vi "Read Com port Name.vi"(11 "Device in":refnum<class "PIC-Device.lvclass">) -> (2 "Com port Name":string, 3 "Device out":refnum<class "PIC-Device.lvclass">)   [LabVIEW 2020, in "PIC-Device.lvclass"]
uses:
  PIC-Device.lvclass
  PIC-Device.lvclass/PIC-Device.ctl
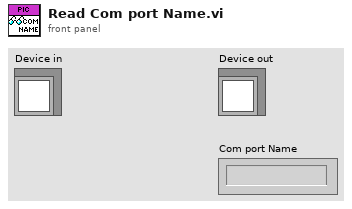
[diagram p1: front panel]
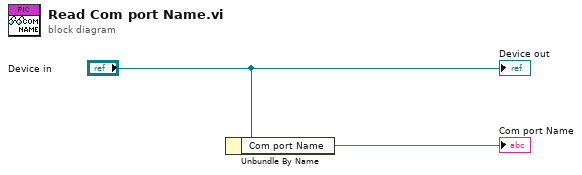
[diagram p0: block diagram]
diagram:
  n1 = Unbundle By Name("Device in") -> ("Com port Name"=→"Com port Name":string)
  "Device out" <- "Device in"
